vi "Button Pressed.vi"(8 "error in (no error)":errorcluster, 9 "action":string, 10 "name":string) -> (0 "error out":errorcluster)   [LabVIEW 2020, in "Navigation.lvlib"]
doc: "Broadcasts the pressed button and optional data.\n____\nHAMPEL SOFTWARE ENGINEERING v2.6.0 (2023-12-19 10:54)"
uses:
  Navigation.lvlib
  Button Pressed Argument--cluster.ctl
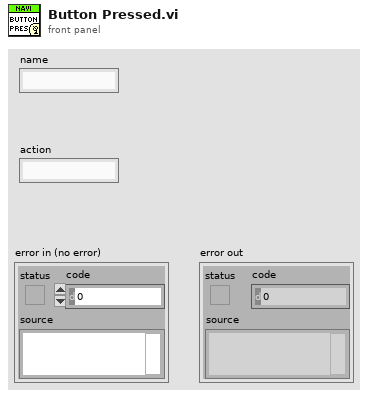
[diagram p1: front panel]
types:
  T1 = typedef "Navigation.lvlib/Button Pressed Argument--cluster.ctl" = cluster{"name":string, "action":string}
  T2 = typedef "Navigation.lvlib/Broadcast Events--cluster.ctl" = cluster{"Module Did Init":refnum<user-event>, "Status Updated":refnum<user-event>, "Error Reported":refnum<user-event>, "Module Did Stop":refnum<user-event>, "Update Module Execution Status":refnum<user-event>, "Button Pressed":refnum<user-event>, "Sub-Control Pressed":refnum<user-event>, "System Message":refnum<user-event>}
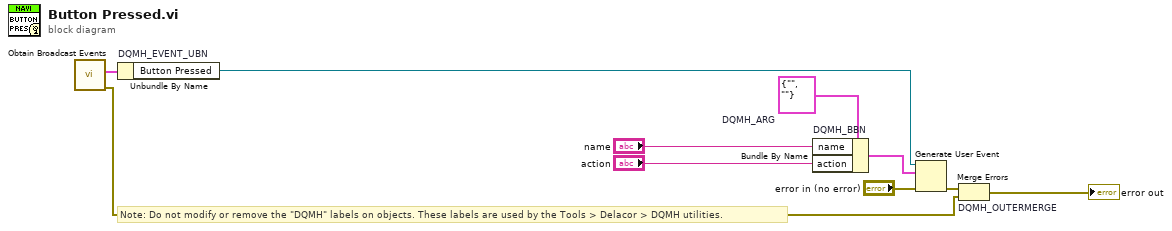
[diagram p0: block diagram]
diagram:
  w5 = T1 {"name"="", "action"=""}  # DQMH_ARG
  # "Note: Do not modify or remove the \"DQMH\" labels on objects. These labels are used by the Tools > Delacor > DQMH utilities."
  n1 = call "Obtain Broadcast Events.vi"() -> ("error out"=w4:errorcluster, "Navigation Broadcast Events"=w3:T2)  [unwired: 10 in]
  n2 = Unbundle By Name "DQMH_EVENT_UBN"(w3) -> ("Button Pressed"=w7:refnum<user-event>)
  n3 = Bundle By Name "DQMH_BBN"(cluster=w5, "name"="name", "action"="action") -> (w8:T1)
  n4 = Generate User Event(user event=w7, event data cluster=w8, error in="error in (no error)") -> (error out=w6:errorcluster)  [unwired: 1 in, 1 out]
  n5 = Merge Errors "DQMH_OUTERMERGE"(w6, w4) -> (→"error out":errorcluster)
